vi "Re-init.vi"(6 "instVIref":T1, 8 "tsRef":refnum<vi>, 11 "target in":refnum<class "Base Target.lvclass">) -> (0 "tsRef out":refnum<vi>, 3 "target out":refnum<class "Base Target.lvclass">)   [LabVIEW 2020, in "NI_TargetHelper.lvlib" / "Base Target.lvclass"]
uses:
  <vilib>/TargetSupport/NI_TargetHelper/Base Target/Base Target.lvclass
  <vilib>/TargetSupport/NI_TargetHelper/Instance VIref.ctl
  24b14142-32ab-4c4f-9960-23eb36978da7.vi
  <vilib>/TargetSupport/NI_TargetHelper/NI_TargetHelper.lvlib
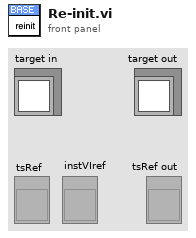
[diagram p1: front panel]
types:
  T1 = typedef "NI_TargetHelper.lvlib/Instance VIref.ctl" = refnum<vi>
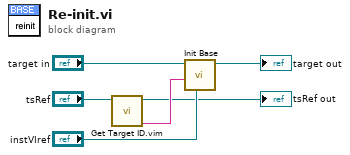
[diagram p0: block diagram]
diagram:
  n1 = call "Get Target ID.vim"("ref in"="tsRef") -> ("target ID"=w3:string, "ref out"=→"tsRef out":refnum<vi>)  [unwired: 9 in]
  n2 = call <vilib>:"Init Base.vi"("instVIref"="instVIref", "target structure name"=w3, "target in"="target in") -> ("target out"=→"target out":refnum<class "Base Target.lvclass">)  [unwired: 8 in]
